vi "KLB Tester.vi"() -> ()   [LabVIEW 2013]
uses:
  File IO/KLB/VIs/Type Defs/KLB Settings Cluster.ctl
  File IO/KLB/VIs/Type Defs/KLB # of CPUs enum.ctl
  File IO/KLB/VIs/Type Defs/KLB compression type enum.ctl
  File IO/KLB/KLB.lvlib
panel:
  in  "Boolean":bool
  out "Images created":i32
  out "klb":i32
  in  "stop":bool
  in  "Path In":path=path "G:/StreamingVideo/test/delete"
  in  "# of Klb":i32=10
  in  "Y":u16=788
  in  "X":u16=1200
  in  "Images per klb":i32=1000
  in  "KLB Settings":T1={"Logical Cores"=enum."CPU 25%", "pixelSize (um)"=[1.0, 1.0, 1.0, 1.0, 1.0], "blockSize"=[384, 192, 1, 1, 1], "compressionType"=enum."BZip2", "metadata"=""} {"pixelSize (um)" min=0.01 max=10 step=0.01 format="%.2f"}
  out "KLB Conversion Time (ms)":u32=53091
  out "error IO":errorcluster
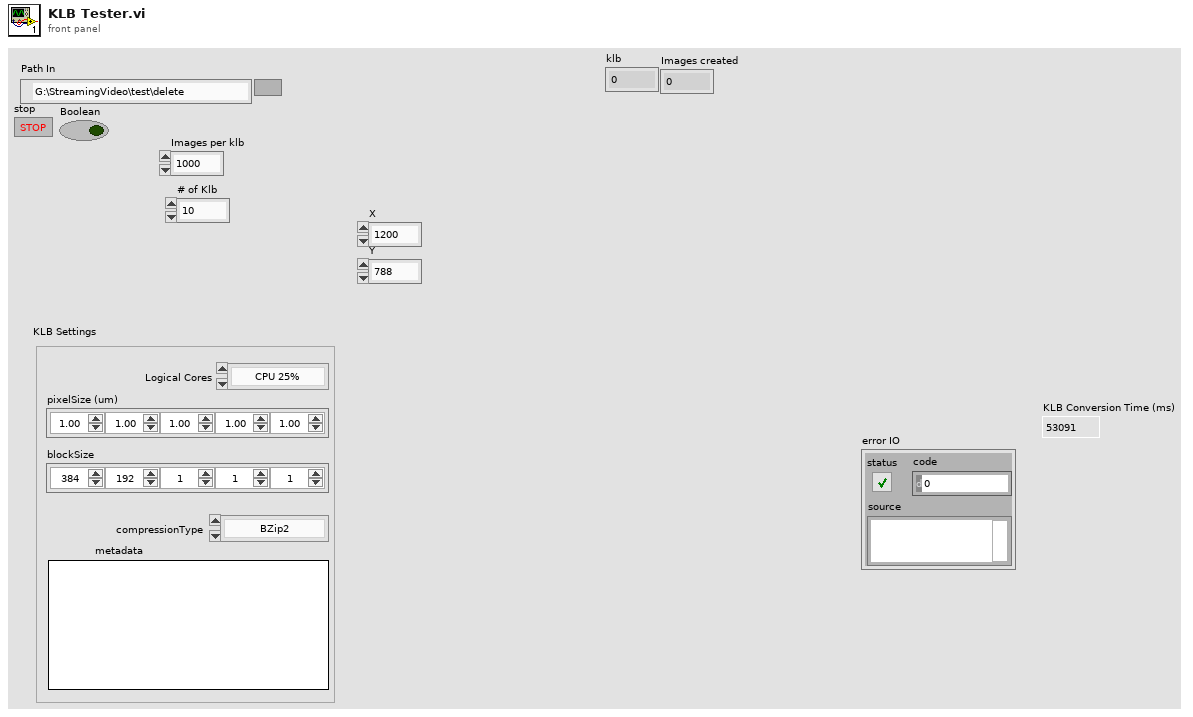
[diagram p1: front panel]
types:
  T1 = typedef "KLB.lvlib/KLB Settings Cluster.ctl" = cluster{"Logical Cores":T2, "pixelSize (um)":sgl[], "blockSize":u32[], "compressionType":T3, "metadata":string}
  T2 = typedef "KLB.lvlib/KLB # of CPUs enum.ctl" = enum16{"CPU 25%", "CPU 50%", "CPU 75%", "CPU All but 1", "1", "4", "8", "16"}
  T3 = typedef "KLB.lvlib/KLB compression type enum.ctl" = enum8{"Uncompressed", "BZip2"}
  T4 = typedef "Image Type" = u32
  T5 = typedef "IMAQ Image.ctl" = refnum<image>
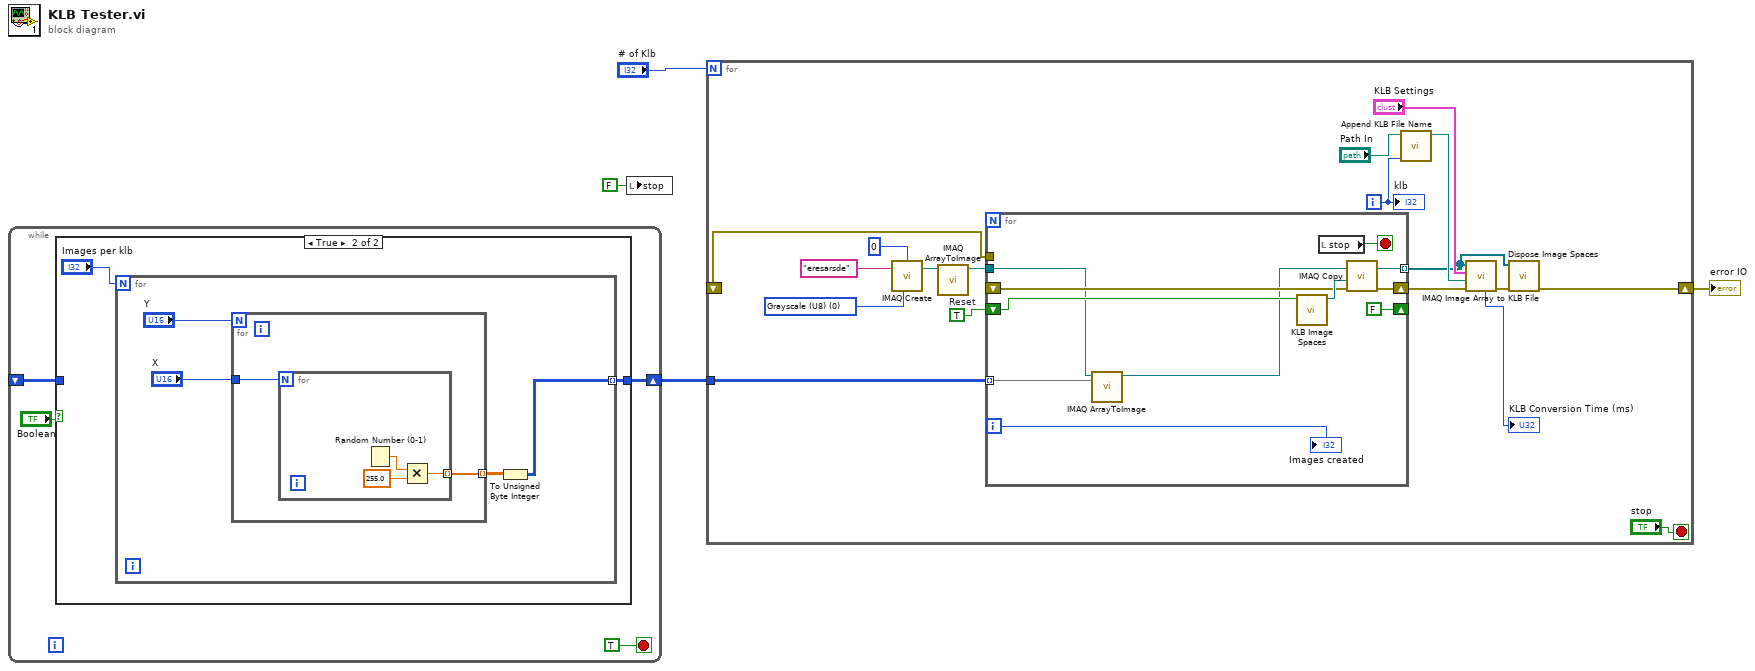
[diagram p0: block diagram]
diagram:
  n1 = while {
    shift-right: [w8] -> w1
    shift-left: _ -> [w5]
    stop <- TRUE stop-if-true
    n2 = case shown="True" "Boolean" {
      tunnel: [w9 w10] -> w8
      tunnel: w5 -> [w9 _]
      frame False {
      }
      frame True {
        n3 = for {
          N: "Images per klb" -> [_]
          tunnel: [w12] -> w10 mode=indexing
          n4 = for {
            N: "Y" -> [_]
            tunnel: "X" -> [w17]
            tunnel: [w16] -> w13 mode=indexing
            n5 = for {
              N: w17 -> [_]
              tunnel: [w18] -> w16 mode=indexing
              n6 = Random Number (0-1)() -> (number: 0 to 1=w19:dbl)
              n7 = Multiply(x=w19, y=255.0) -> (x*y=w18:dbl)
            }
          }
          n8 = To Unsigned Byte Integer(number=w13) -> (unsigned 8bit integer=w12:u8[][])
        }
      }
    }
  }
  n9 = local write "stop"(FALSE ("stop")) -> ()
  n10 = for {
    N: "# of Klb" -> [_]
    shift-right: [w28] -> w3
    shift-left: _ -> [w27]
    tunnel: w1 -> [w21]
    i -> [w33]
    stop <- "stop" stop-if-true
    w23 = T4 0 items=["Grayscale (U8)", "Grayscale (I16)", "Grayscale (SGL)", "Complex (CSG)", "RGB (U32)", "HSL (U32)", "RGB (U64)", "Grayscale (U16)"] ("Image Type")
    w34 = TRUE  # Reset
    n11 = call "IMAQ Create"("Border Size"=0, "Image Name"="eresarsde", "Image Type"=w23) -> ("New Image"=w25:T5)  [unwired: 2 in, 1 out]
    n12 = call "IMAQ ArrayToImage"("Image"=w25) -> ("Image Out"=w22:T5)  [unwired: 9 in, 1 out]
    n13 = for {
      shift-right: [FALSE ("Reset")] -> _
      shift-left: w34 -> [w49]
      tunnel: w27 -> [_]
      tunnel: [w46] -> w29 mode=indexing
      shift-right: [w44] -> w31
      shift-left: _ -> [w45]
      tunnel: w22 -> [w40]
      tunnel: w21 -> [w41] mode=indexing
      i -> [w42]
      stop <- w43 stop-if-true
      n14 = call "IMAQ ArrayToImage"("Image Pixels (U8)"=w41, "Image"=w40) -> ("Image Out"=w39:T5)  [unwired: 8 in, 1 out]
      n15 = call "KLB Image Spaces.vi"("Reset?"=w49) -> ("U8 Image"=w47:T5)  [unwired: 8 in, 2 out]
      n16 = local read "stop"() -> (w43:bool)
      n17 = call "IMAQ Copy"("error in (no error)"=w45, "Image Dst"=w47, "Image Src"=w39) -> ("error out"=w44:errorcluster, "Image Dst Out"=w46:T5)  [unwired: 3 in]
      "Images created" <- w42
    }
    n18 = call "Append KLB File Name.vi"("Iteration"=w33, "Path In"="Path In") -> ("Path Out"=w36:path)  [unwired: 9 in]
    n19 = call "IMAQ Image Array to KLB File.vi"("error in (no error)"=w31, "path"=w36, "KLB Settings"="KLB Settings", "Images to Compress"=w29) -> ("error out"=w30:errorcluster, "elapsed (ms)"=→"KLB Conversion Time (ms)":u32)  [unwired: 6 in]
    n20 = call "Dispose Image Spaces.vi"("error in (no error)"=w30, "[Images]"=w29) -> ("error out"=w28:errorcluster)  [unwired: 9 in]
    "klb" <- w33
  }
  "error IO" <- w3
